vi "PythonName.vi"(6 "add self":bool=TRUE, 8 "error in":errorcluster, 11 "GObject in":refnum<class "GObject.lvclass">) -> (0 "error out":errorcluster, 3 "GObject out":refnum<class "GObject.lvclass">, 5 "name":string, 7 "UID":string)   [LabVIEW 2014, in "Raspberry Pi Compatible Compiler for LabVIEW.lvlib" / "GObject.lvclass"]
uses:
  GObject.lvclass
  Python/Parsing/Python Functions.lvlib
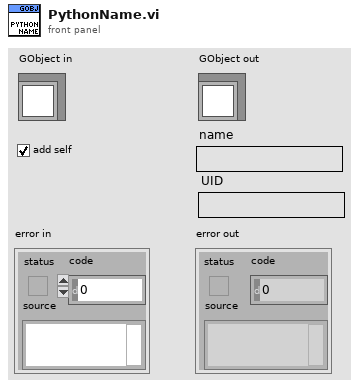
[diagram p1: front panel]
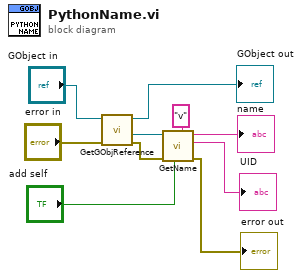
[diagram p0: block diagram]
diagram:
  n1 = call "GetGObjReference.vi"("error in"="error in", "GObject in"="GObject in") -> ("error out"=w8:errorcluster, "reference out"=w9:refnum<vi>, "GObject out"=→"GObject out":refnum<class "GObject.lvclass">)  [unwired: 5 in]
  n2 = call "GetName.vi"("base name"="v", "add self"="add self", "error in"=w8, "GObj Refnum"=w9) -> ("error out"=→"error out":errorcluster, "UID"=→"UID":string, "name"=→"name":string)  [unwired: 5 in]
